vi "get_acceleration.vi"(8 "error in (no error)":errorcluster, 11 "Picomotor in":refnum<class "Picomotor.lvclass">) -> (0 "error out":errorcluster, 2 "Acceleration (steps/sec^2)":dbl, 3 "Picomotor out":refnum<class "Picomotor.lvclass">)   [LabVIEW 2020, in "Picomotor.lvclass"]
uses:
  Picomotor.lvclass
  Picomotor.lvclass/Picomotor.ctl
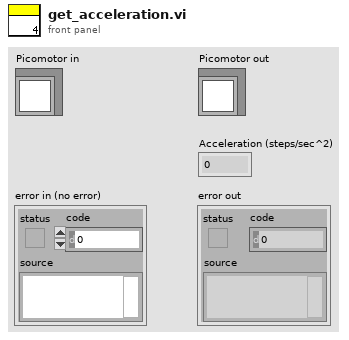
[diagram p1: front panel]
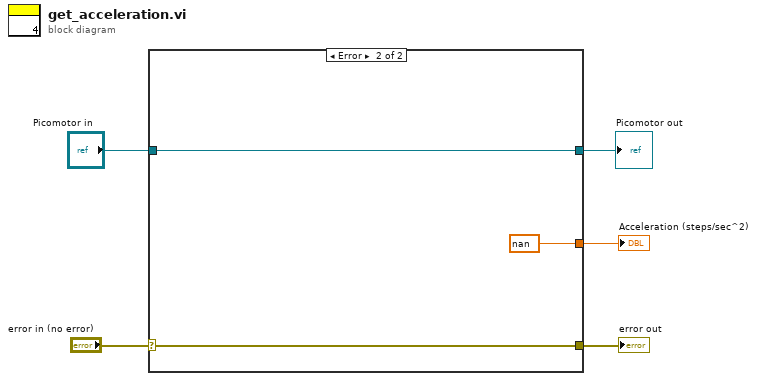
[diagram p0: block diagram]
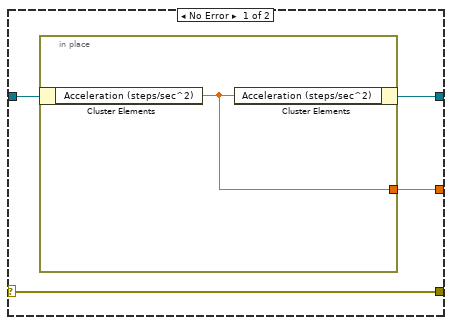
[diagram p2: hidden frame]
diagram:
  n1 = case shown="Error" "error in (no error)" {
    selector: "error in (no error)" -> [w9 w13]
    tunnel: [w9 w13] -> w4
    tunnel: [w7 w12] -> w2
    tunnel: "Picomotor in" -> [w8 w12]
    tunnel: [w6 nan] -> w1
    frame No Error {
      n2 = in-place {
        in-place-border: [w10] -> w6
        n3 = in-place-cluster #1(w8) -> ("Acceleration (steps/sec^2)"=w10:dbl)
        n4 = in-place-cluster #1("Acceleration (steps/sec^2)"=w10) -> (w7:refnum<class "Picomotor.lvclass">)
      }
    }
    frame Error {
    }
  }
  "error out" <- w4
  "Picomotor out" <- w2
  "Acceleration (steps/sec^2)" <- w1
